vi "Galobal variable_TI.vi"() -> ()   [LabVIEW 2015]
panel:
  out "Operator code":string
  in  "Server":bool
  in  "Shift":T1
  in  "Rework Bit":bool
  out "Tracibility":bool
  out "Pokayoka Status":bool
  in  "NG Count":u8
  in  "Shift  Change":string
  in  "User ID":string
  in  "Rpt Read":bool
  in  "Rpt Write":bool
  in  "Safety Inte. I/o":bool
  out "Actuator2-Offset":dbl
  out "Actuator1-Offset":dbl
  out "Camera communication":bool
  in  "Trigger":bool
  out "Error color bit":bool
  out "Load OFFSET":dbl
  in  "Load Trigger Bit":bool
  in  "Load Trigger bit":bool
  out "Load Data":dbl
  out "Lvdt &Load Result":T2 {"Load(N)" format="%0.02f"; "Actuator1(mm)" format="%0.02f"; "Actuator2(mm)" format="%0.02f"}
  out "Load & Lvdt data":T3
  out "Error color":u32
  in  "Cam write data":string
  in  "Model  Triger bit 2":bool
  in  "Camera Triger bit":bool
  in  "Co-ordinate":string
  out "Camera NG":bool
  out "Camera Ok":bool
  in  "MIC Barcode":string="0UD6I20MUW7W"
  in  "LCD Barcode":string
  in  "Barcode Setting":T4={"MIC "="COM2", "baud rate MIC "=115200, "LCD "="COM1", "baud rate_LCD"=115200}
  out "IL Sensor_Pokayoka":bool[](array[boolean])
  in  "Running Model":string
  in  "Sensor Setting Data":T5
  out "Sensor Data":T6
  in  "NI Comm.Error":bool
  in  "LVDT":dbl format="%0.03f"
  in  "Load Cell":dbl format="%0.03f"
  in  "Digital Output":bool[](array[boolean])
  in  "Auto Exit":bool
  in  "Slid Servo Home bit":bool
  in  "Call Home M2":bool
  in  "Call Home M1":bool
  in  "Barcode Lenght":i32
  in  "Barcode Scan Bit":bool
  in  "Barcode Data":string
  in  "Control Enable":bool
  in  "Stop M1":bool
  in  "Stop M2":bool
  in  "Programlist":string[](array[string])
  in  "STM Done Bit":bool
  in  "Offset_2":dbl
  in  "Offset_1":dbl
  in  "Slop _2":dbl
  in  "Slop_1":dbl
  out "Analoge Input":dbl[](array[numeric])
  out "AI_as DI":bool[](array[boolean])
  out "Manual DO":bool[](array[boolean])
  in  "Manual CMD":bool
  out "File Path":path[](array[path])
  out "Digital input":bool[](array[boolean])
  in  "User Name":string
  in  "Exit":bool
  # "LOAD DATA"
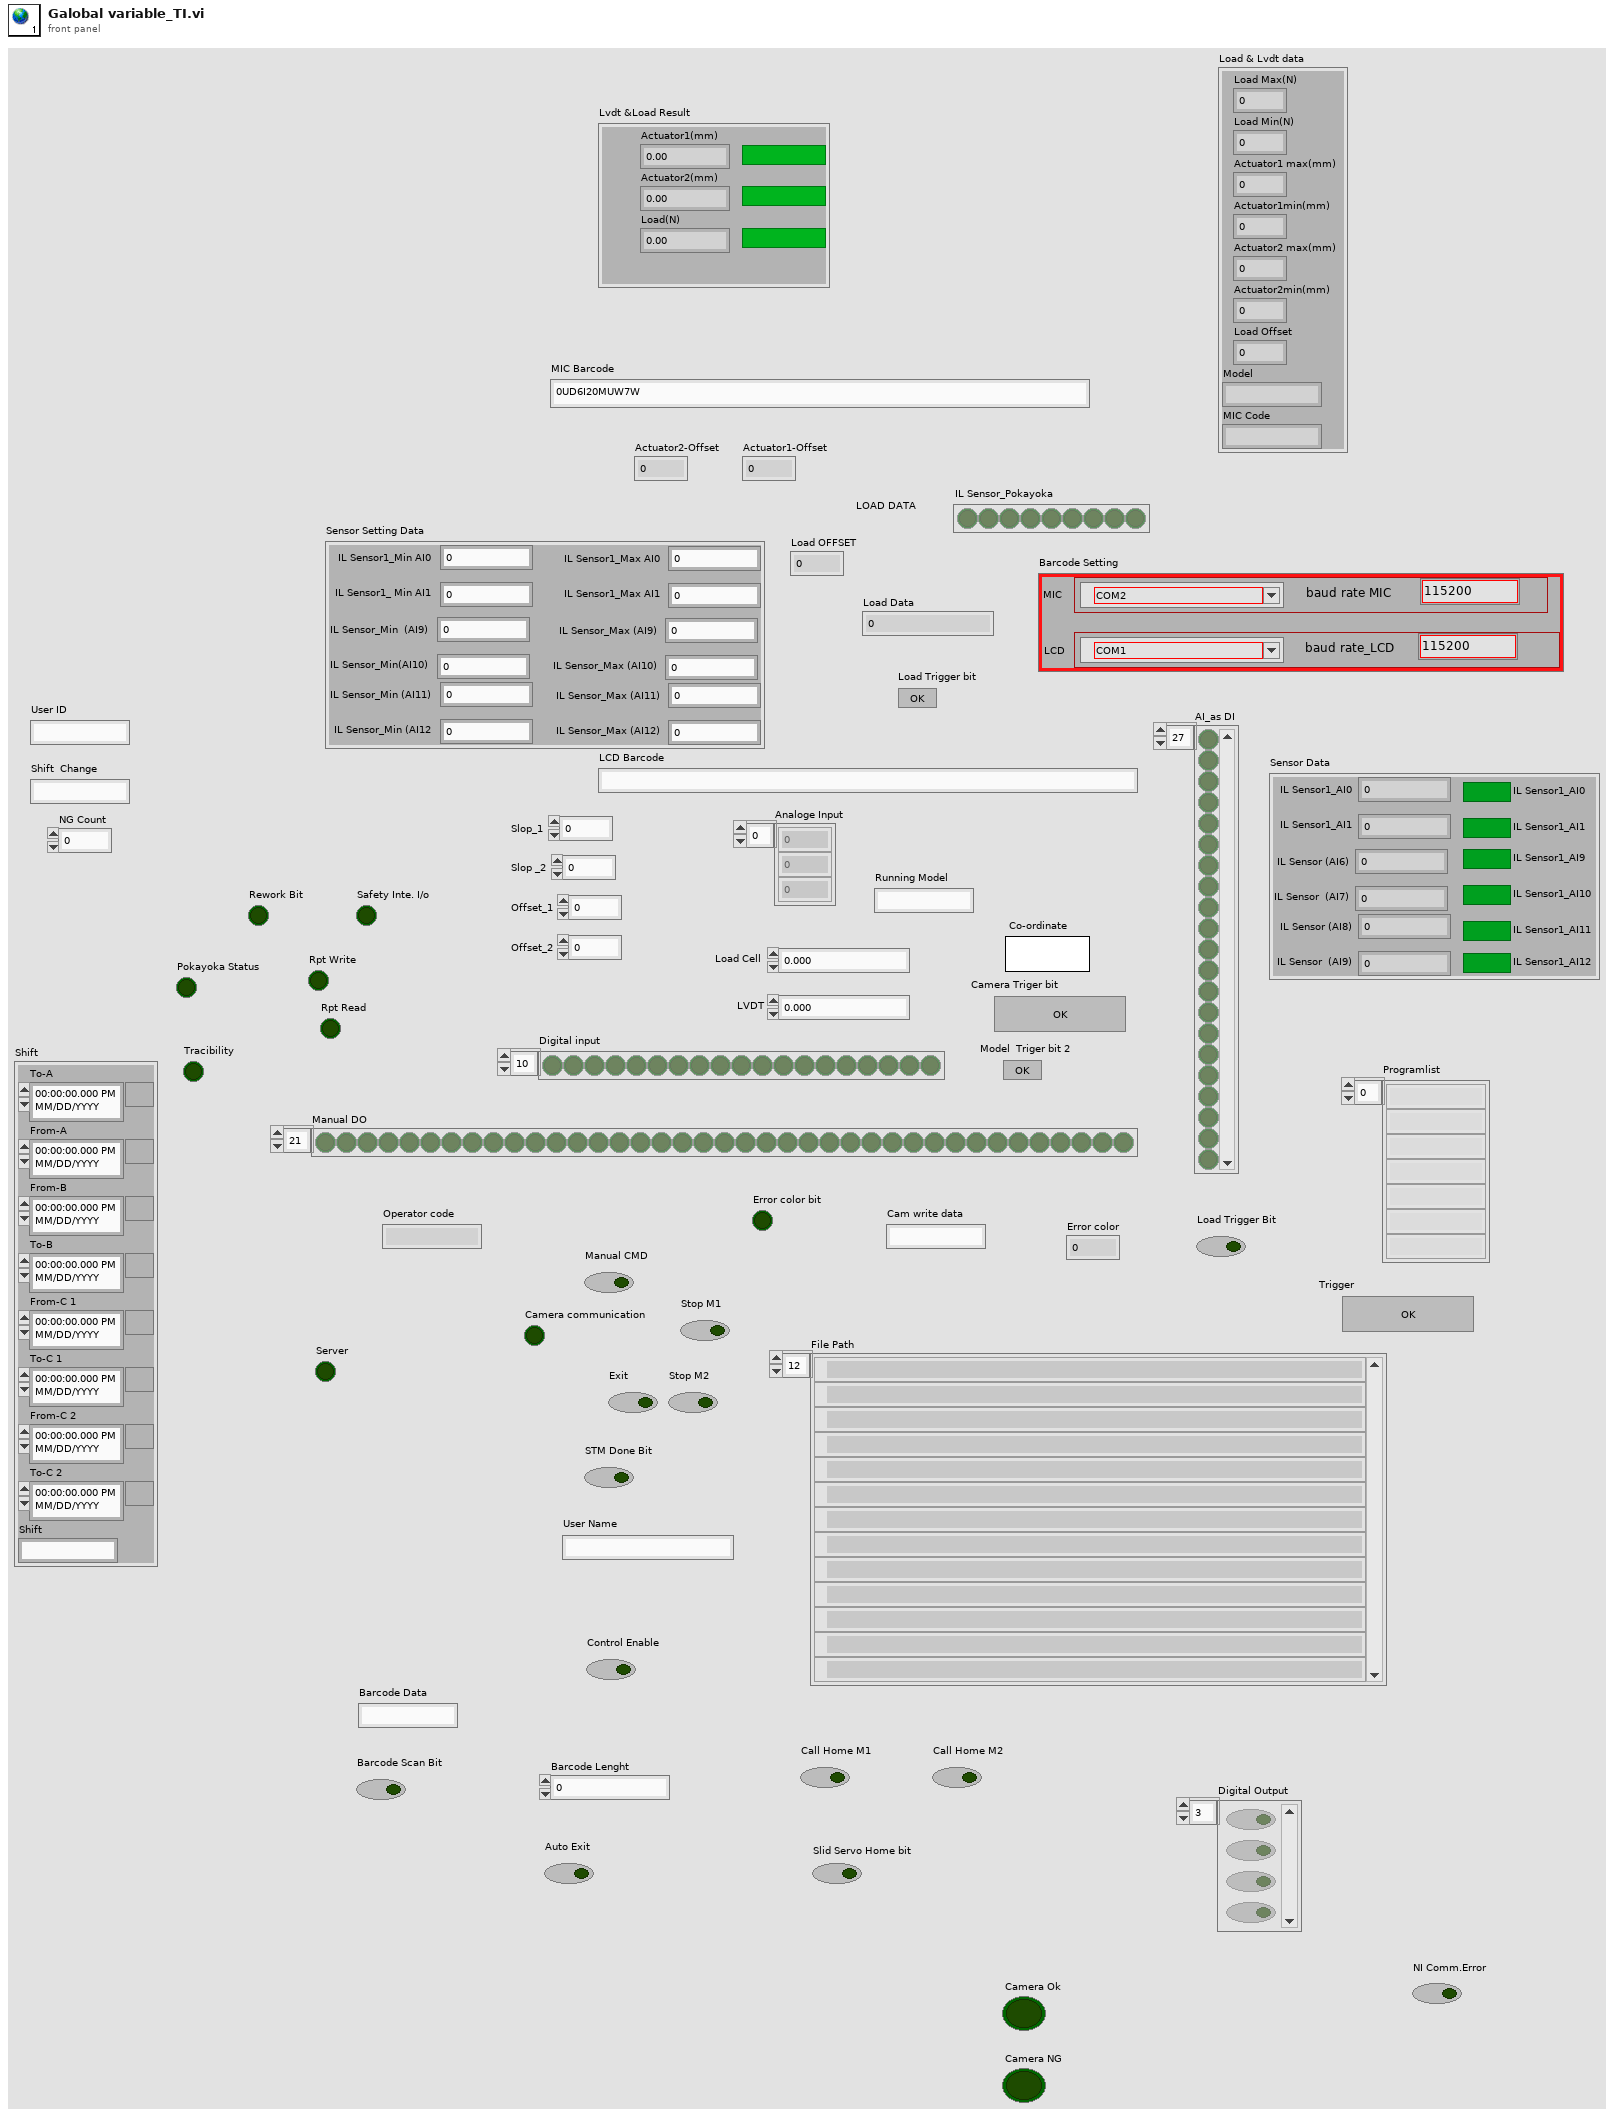
[diagram p1: front panel]
types:
  T1 = cluster{"To-A":timestamp, "From-A":timestamp, "From-B":timestamp, "To-B":timestamp, "From-C 1":timestamp, "To-C 1":timestamp, "From-C 2":timestamp, "To-C 2":timestamp, "Shift":string}
  T2 = cluster{"Actuator1(mm)":dbl, "Actuator2(mm)":dbl, "Load(N)":dbl, "Actuator1":bool, "Actuator2":bool, "Load":bool}
  T3 = cluster{"Load Max(N)":dbl, "Load Min(N)":dbl, "Actuator1 max(mm)":dbl, "Actuator1min(mm)":dbl, "Actuator2 max(mm)":dbl, "Actuator2min(mm)":dbl, "Load Offset":dbl, "Model":string, "MIC Code":string}
  T4 = cluster{"MIC ":refnum<visa-resource-name>, "baud rate MIC ":u32, "LCD ":refnum<visa-resource-name>, "baud rate_LCD":u32}
  T5 = cluster{"IL Sensor1_Max AI0":dbl, "IL Sensor1_Min AI0":dbl, "IL Sensor1_Max AI1":dbl, "IL Sensor1_ Min AI1":dbl, "IL Sensor_Max (AI9)":dbl, "IL Sensor_Min  (AI9)":dbl, "IL Sensor_Max (AI10)":dbl, "IL Sensor_Min(AI10)":dbl, "IL Sensor_Max (AI11)":dbl, "IL Sensor_Min (AI11)":dbl, "IL Sensor_Max (AI12)":dbl, "IL Sensor_Min (AI12":dbl}
  T6 = cluster{"IL Sensor1_AI0":dbl, "IL Sensor1_AI1":dbl, "IL Sensor (AI6)":dbl, "IL Sensor  (AI7)":dbl, "IL Sensor (AI8)":dbl, "IL Sensor  (AI9)":dbl, "IL Sensor1_AI0":bool, "IL Sensor1_AI1":bool, "IL Sensor1_AI9":bool, "IL Sensor1_AI10":bool, "IL Sensor1_AI11":bool, "IL Sensor1_AI12":bool}
diagram:
